vi "FL3001_simpleFFT.VI"() -> ()   [LabVIEW 2015]
uses:
  board.vis/Globals.vi
panel:
  in  "continuous":bool
  in  "exit":bool
  out "meanB":dbl=197.0 format="%0#.1f"
  out "tRMSB":dbl format="%0#.1f"
  out "meanA":dbl=9163.524137931034 format="%0#.1f"
  in  "TRMS Pix":u32=550
  out "Signal Cam 2":u16[](graph)
  in  "extTrig":bool
  in  "ext. trig. slope":enum32{"1", "2", "3"}(radio)
  out "tRMSA":dbl=7.44979324293522 format="%0#.1f"
  out "Measure ON":bool
  in  "no.of blocks (nob)":u32=1
  in  "block":u32(slide)=1 max=10 scale=0.9..1.0
  out "Signal Cam1":u16[](graph)=[9561, 9604, 0, 1, 0, 328, 0, 0, 9709, 10494, 10571, 10581, 10601, 10615, 10647, 10653, 10690, 10710, 10746, 10759, 10759, 10759, 10895, 10918, 10956, 10990, 11009, 11035, 11062, 11093, 11094, 11132, 11153, 11163, 11174, 11214, 11226, 11266, 11275, 11312, 11312, 11332, 11366, 11390, 11417, 11427, 11449, 11469, 11521, 11534, 11583, 11593, 11641, 11662, 11679, 11694, 11737, 11762, 11774, 11783, 11783, 11783, 11783, 11783, 11920, 11930, 11959, 11974, 11989, 12026, 12049, 12084, 12103, 12150, 12155, 12183, 12211, 12240, 12248, 12284, 12315, 12354, 12370, 12377, 12400, 12438, 12452, 12496, 12508, 12527, 12549, 12602, 12594, 12642, 12656, 12681, 12709, 12743, 12757, 12795, 12794, 12807, 12807, 12807, 12807, 12807, 12807, 12967, 12988, 13001, 13011, 13047, 13089, 13091, 13092, 13129, 13161, 13146, 13209, 13224, 13248, 13291, 13287, 13299, 13340, 13369, 13392, 13408, 13438, 13466, 13473, 13527, 13541, 13568, 13587, 13627, 13657, 13707, 13731, 13760, 13817, 13831, 13831, 13831, 13831, 13989, 14036, 14106, 14146, 14191, 14230, 14290, 14338, 14392, 14441, 14483, 14518, 14577, 14638, 14699, 14740, 14794, 14855, 14855, 14855, 15072, 15093, 15168, 15231, 15307, 15358, 15391, 15480, 15534, 15615, 15686, 15769, 15819, 15891, 15968, 16012, 16100, 16195, 16252, 16337, 16412, 16476, 16563, 16632, 16689, 16784, 16856, 16903, 16903, 17060, 17153, 17223, 17287, 17387, 17454, 17529, 17634, 17720, 17787, 17874, 17927, 17927, 18168, 18238, 18341, 18440, 18540, 18602, 18704, 18811, 18897, 18951, 19096, 19210, 19315, 19399, 19518, 19623, 19758, 19826, 19927, 19975, 19975, 20226, 20347, 20459, 20564, 20669, 20798, 20885, 20999, 21131, 21240, 21332, 21432, 21582, 21689, 21801, 21933, 22036, 22143, 22221, 22353, 22440, 22547, 22624, 22719, 22796, 22893, 22979, 23047, 23047, 23208, 23319, 23398, 23462, 23562, 23613, 23731, 23808, 23873, 23975, 24037, 24071, 24071, 24296, 24399, 24443, 24531, 24616, 24700, 24811, 24871, 24952, 25035, 25093, 25248, 25309, 25404, 25478, 25546, 25615, 25718, 25827, 25902, 25997, 26044, 26119, 26119, 26323, 26393, 26479, 26574, 26649, 26720, 26792, 26910, 27011, 27074, 27143, 27143, 27350, 27420, 27510, 27599, 27681, 27712, 27801, 27905, 28024, 28110, 28167, 28167, 28345, 28409, 28433, 28482, 28469, 28507, 28495, 28432, 28406, 28317, 28167, 28167, 28037, 27914, 27802, 27663, 27539, 27380, 27143, 27046, 26887, 26742, 26596, 26445, 26310, 26119, 26009, 25909, 25785, 25678, 25595, 25531, 25422, 25393, 25361, 25332, 25299, 25313, 25357, 25399, 25446, 25511, 25518, 25660, 25718, 25827, 25907, 25944, 25898, 25886, 25845, 25777, 25728, 25600, 25541, 25445, 25348, 25245, 25095, 25024, 24905, 24756, 24560, 24358, 24071, 23885, 23654, 23369, 23047, 22894, 22611, 22355, 22091, 21833, 21605, 21356, 21137, 20900, 20682, 20479, 20244, 19975, 19822, 19604, 19367, 19176, 18932, 18710, 18477, 18257, 17927, 17833, 17611, 17395, 17228, 16903, 16883, 16696, 16542, 16398, 16249, 16123, 15993, 15866, 15774, 15655, 15547, 15463, 15391, 15336, 15264, 15207, 15179, 15158, 15112, 15116, 15127, 15136, 15151, 15158, 15184, 15215, 15229, 15210, 15261, 15273, 15277, 15302, 15311, 15315, 15328, 15351, 15344, 15367, 15377, 15392, 15403, 15438, 15408, 15430, 15451, 15463, 15452, 15449, 15470, 15507, 15491, 15503, 15522, 15535, 15543, 8347, 8048, 8032, 8045, 8044, 8055, 8082, 8087, 8108, 8111, 8134, 8143, 8159, 8166, 8186, 8194, 8224, 8225, 8237, 8257, 8266, 8278, 8305, 8318, 8318, 8340, 8348, 8366, 8366, 8394, 8406, 8411, 8434, 8457, 8461, 8478, 8488, 8508, 8518, 8526, 8552, 8559, 8577, 8583, 8591, 8616, 8627, 8644, 8664, 8676, 8698, 8711, 8711, 8711, 8711, 8711, 8711, 8711, 8711, 8711, 8853, 8863, 8888, 8902, 8896, 8922, 8938, 8959, 8969, 8991, 9002, 9022, 9040, 9048, 9060, 9086, 9098, 9104, 9137, 9153, 9161, 9169, 9180, 9193, 9203, 9221, 9241, 9252, 9251, 9281, 9300, 9303, 9324, 9351, 9344, 9362, 9383, 9395, 9430, 9442, 9447, 9464, 9490, 9513, 9522, 9532, 9564]
  out "FREE \nRAM MB":dbl=27108.19140625
  out "BUILT-IN\nRAM MB":dbl=32640.29296875
  out "SEC":dbl=0.5
  out "MB RAM":dbl=0.54931640625
  in  "DAT in 10ns":u32
  in  "start":bool
  in  "sample":u32(slide)=328 max=3000 scale=0.9..500.0
  in  "no.of samples (nos)":u32=500
  in  "exposuretime[ms]":dbl=1.0 format="%.3f"
  # "press cont to stop, \nEsc to abort\nmeasurement"
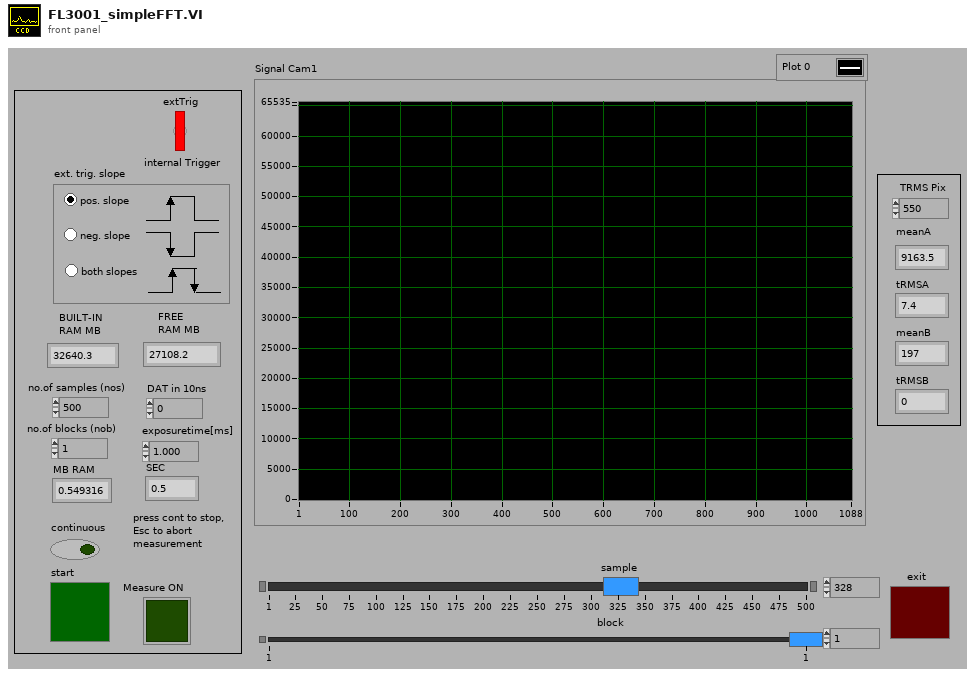
[diagram p1: front panel]
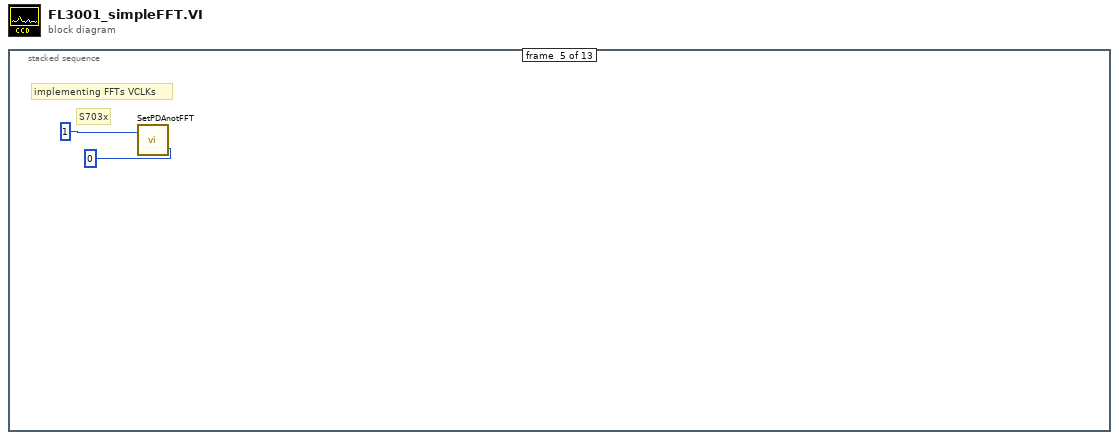
[diagram p0: block diagram]
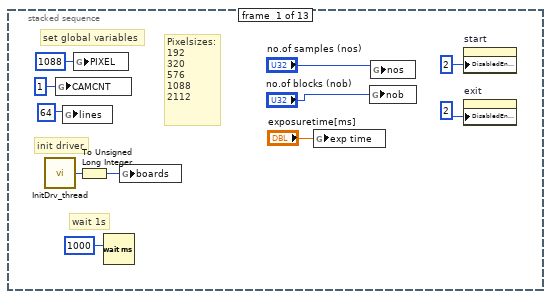
[diagram p2: hidden frame]
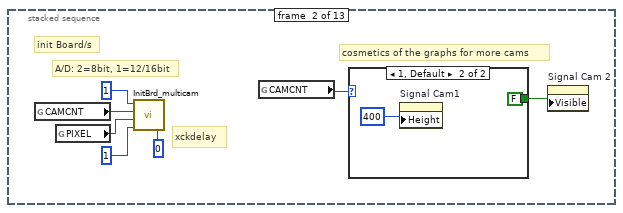
[diagram p3: hidden frame]
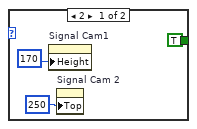
[diagram p4: hidden frame]
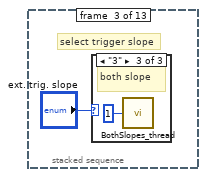
[diagram p5: hidden frame]
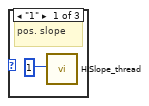
[diagram p6: hidden frame]
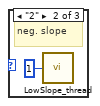
[diagram p7: hidden frame]
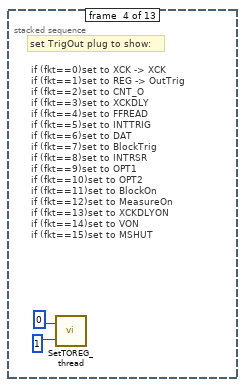
[diagram p8: hidden frame]
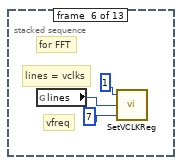
[diagram p9: hidden frame]
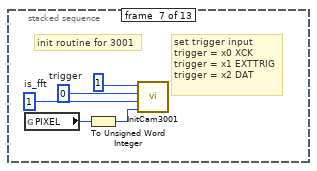
[diagram p10: hidden frame]
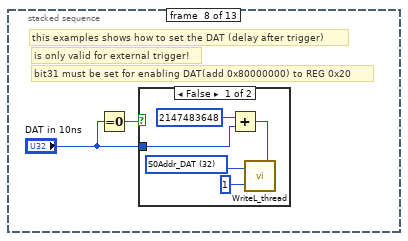
[diagram p11: hidden frame]
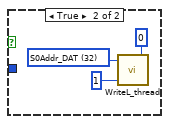
[diagram p12: hidden frame]
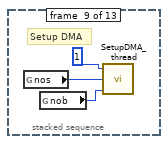
[diagram p13: hidden frame]
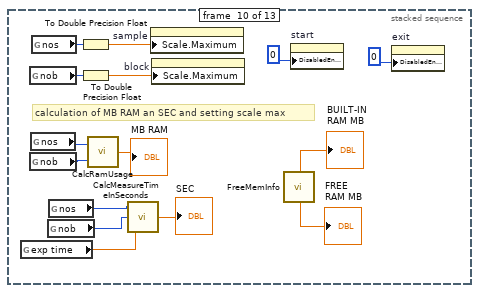
[diagram p14: hidden frame]
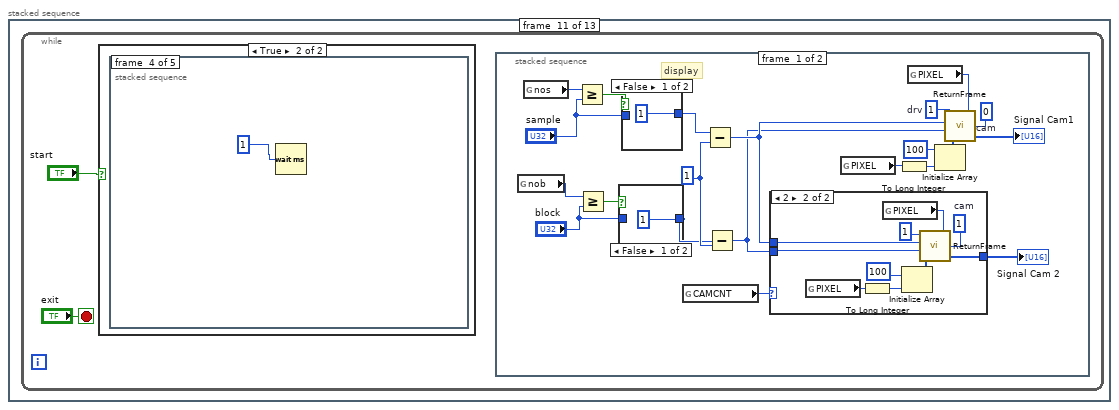
[diagram p15: hidden frame]
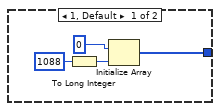
[diagram p16: hidden frame]
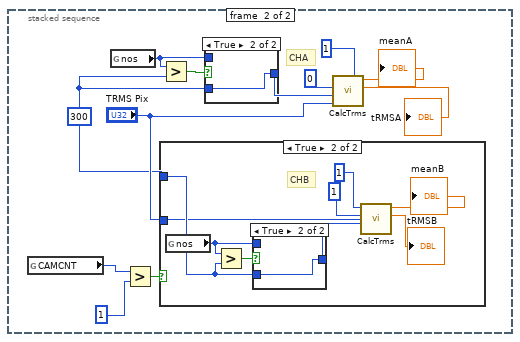
[diagram p19: hidden frame]
diagram:
  n1 = stacked-sequence {
    frame #0 {
      # "wait 1s"
      # "Pixelsizes:\n192\n320\n576\n1088\n2112"
      # "set global variables"
      # "init driver"
      n2 = call "InitDrv_thread.vi"() -> ("Boards"=w11:u8)  [unwired: 1 in]
      n3 = global write "Globals.vi" "CAMCNT"(u32 1) -> ()
      n4 = global write "Globals.vi" "lines"(u32 64) -> ()
      n5 = global write "Globals.vi" "PIXEL"(u32 1088) -> ()
      n6 = To Unsigned Long Integer(number=w11) -> (unsigned 32bit integer=w10:u32)
      n7 = Wait (ms)(milliseconds to wait=u32 1000) -> ()  [unwired: 1 out]
      n8 = global write "Globals.vi" "boards"(w10) -> ()
      n9 = global write "Globals.vi" "exp time"("exposuretime[ms]") -> ()
      n10 = global write "Globals.vi" "nob"("no.of blocks (nob)") -> ()
      n11 = global write "Globals.vi" "nos"("no.of samples (nos)") -> ()
      n12 = property on="start" class="Bool (strict)"("DisabledEnum"=u32 2) -> ()  [unwired: 2 in, 2 out]
      n13 = property on="exit" class="Bool (strict)"("DisabledEnum"=u32 2) -> ()  [unwired: 2 in, 2 out]
    }
    frame #1 {
      # "cosmetics of the graphs for more cams"
      # "xckdelay"
      # "init Board/s"
      # "A/D: 2=8bit, 1=12/16bit"
      n14 = global read "Globals.vi" "CAMCNT"() -> (w18:u32)
      n15 = global read "Globals.vi" "PIXEL"() -> (w16:u32)
      n16 = call "InitBrd_multicam.vi"("xckdly"=u32 0, "flag816"=u32 1, "pixel"=w16, "camcnt"=w18, "board_sel"=u32 1) -> ()  [unwired: 2 in]
      n17 = global read "Globals.vi" "CAMCNT"() -> (w12:u32)
      n18 = case shown="1, Default" w12 {
        tunnel: [TRUE FALSE] -> w13
        frame 2 {
          n19 = property on="Signal Cam1" class="WFGraph (strict)"("Height"=u32 170) -> ()  [unwired: 2 in, 2 out]
          n20 = property on="Signal Cam 2" class="WFGraph (strict)"("Top"=250) -> ()  [unwired: 2 in, 2 out]
        }
        frame 1, Default {
          n21 = property on="Signal Cam1" class="WFGraph (strict)"("Height"=u32 400) -> ()  [unwired: 2 in, 2 out]
        }
      }
      n22 = property on="Signal Cam 2" class="WFGraph (strict)"("Visible"=w13) -> ()  [unwired: 2 in, 2 out]
    }
    frame #2 {
      # "select trigger slope"
      n23 = case shown="\"3\"" "ext. trig. slope" {
        frame "1" {
          # "pos. slope"
          n24 = call "HiSlope_thread.vi"("board_sel"=u32 1) -> ()  [unwired: 1 in]
        }
        frame "2" {
          # "neg. slope"
          n25 = call "LowSlope_thread.vi"("board_sel"=u32 1) -> ()  [unwired: 1 in]
        }
        frame "3" {
          # "both slope"
          n26 = call "BothSlopes_thread.vi"("board_sel"=u32 1) -> ()  [unwired: 1 in]
        }
      }
    }
    frame #3 {
      # "if (fkt==0)set to XCK -> XCK\nif (fkt==1)set to REG -> OutTrig\nif (fkt==2)set to CNT_O\nif (fkt==3)set to XCKDLY\nif (fkt==4)set to FFREAD\nif (fkt==5)set to INTTRIG\nif (fkt==6)set to DAT\nif (fkt==7)set to BlockTrig\nif (fkt==8)set to INTRSR\nif (fkt==9)set to OPT1\nif (fkt==10)set to OPT2\nif (fkt==11)set to BlockOn\nif (fkt==12)set to MeasureOn\nif (fkt==13)set to XCKDLYON \nif (fkt==14)set to VON         \nif (fkt==15)set to MSHUT"
      # "set TrigOut plug to show:"
      n27 = call "SetTOREG_thread.vi"("board_sel"=u32 1, "fkt"=u8 0) -> ()  [unwired: 1 in]
    }
    frame #4 {
      # "S703x"
      # "implementing FFTs VCLKs"
      n28 = call "SetPDAnotFFT.vi"("set"=u8 0, "board_sel"=u32 1) -> ()  [unwired: 1 in]
    }
    frame #5 {
      # "vfreq"
      # "lines = vclks"
      # "for FFT"
      n29 = global read "Globals.vi" "lines"() -> (w34:u32)
      n30 = call "SetVCLKReg.vi"("vfreq"=u8 7, "lines"=w34, "board_sel"=u32 1) -> ()  [unwired: 1 in]
    }
    frame #6 {
      w35 = u16 1  # is_fft
      w36 = u16 0  # trigger
      # "set trigger input\ntrigger = x0 XCK\ntrigger = x1 EXTTRIG\ntrigger = x2 DAT"
      # "init routine for 3001"
      n31 = global read "Globals.vi" "PIXEL"() -> (w39:u32)
      n32 = To Unsigned Word Integer(number=w39) -> (unsigned 16bit integer=w37:u16)
      n33 = call "InitCam3001.vi"("pixel"=w37, "IS_FFT"=w35, "trigger_input"=w36, "drvno"=u32 1) -> ()  [unwired: 1 in]
    }
    frame #7 {
      # "bit31 must be set for enabling DAT(add 0x80000000) to REG 0x20"
      # "is only valid for external trigger!"
      # "this examples shows how to set the DAT (delay after trigger)"
      n34 = Equal To 0?(x="DAT in 10ns") -> (x = 0?=w41:bool)
      n35 = case shown="False" w41 {
        tunnel: "DAT in 10ns" -> [w45 _]
        frame False {
          w43 = u8 32 items=["S0Addr_CtrlA"=4, "S0Addr_CtrlB"=5, "S0Addr_CtrlC"=6, "S0Addr_XCKLL"=8, "S0Addr_XCKLH"=9, "S0Addr_XCKHL"=10, "S0Addr_XCKMSB"=11, "S0Addr_XCKCNTLL"=12, "S0Addr_XCKCNTLH"=13, "S0Addr_XCKCNTHL"=14, "S0Addr_XCKCNTMSB"=15, "S0Addr_PIXREGlow"=16, "S0Addr_PIXREGhigh"=17, "S0Addr_FREQREG"=18, "S0Addr_FF_FLAGS"=19, "S0Addr_FIFOCNT"=20, "S0Addr_VCLKCTRL"=24, "S0Addr_EBST"=28, "S0Addr_DAT"=32, "S0Addr_EC"=36, "S0Addr_TOR"=40, "S0Addr_ARREG"=44, "S0Addr_GIOREG"=48, "S0Addr_DELAYEC"=52, "S0Addr_IRQREG"=56, "S0Addr_PCI"=60]
          n36 = Add(x=u32 2147483648, y=w45) -> (x+y=w44:u32)
          n37 = call "WriteL_thread.vi"("val"=w44, "board_sel"=u32 1, "offset"=w43) -> ()
        }
        frame True {
          w48 = u8 32 items=["S0Addr_CtrlA"=4, "S0Addr_CtrlB"=5, "S0Addr_CtrlC"=6, "S0Addr_XCKLL"=8, "S0Addr_XCKLH"=9, "S0Addr_XCKHL"=10, "S0Addr_XCKMSB"=11, "S0Addr_XCKCNTLL"=12, "S0Addr_XCKCNTLH"=13, "S0Addr_XCKCNTHL"=14, "S0Addr_XCKCNTMSB"=15, "S0Addr_PIXREGlow"=16, "S0Addr_PIXREGhigh"=17, "S0Addr_FREQREG"=18, "S0Addr_FF_FLAGS"=19, "S0Addr_FIFOCNT"=20, "S0Addr_VCLKCTRL"=24, "S0Addr_EBST"=28, "S0Addr_DAT"=32, "S0Addr_EC"=36, "S0Addr_TOR"=40, "S0Addr_ARREG"=44, "S0Addr_GIOREG"=48, "S0Addr_DELAYEC"=52, "S0Addr_IRQREG"=56, "S0Addr_PCI"=60]
          n38 = call "WriteL_thread.vi"("val"=u32 0, "board_sel"=u32 1, "offset"=w48) -> ()
        }
      }
    }
    frame #8 {
      # "Setup DMA"
      n39 = global read "Globals.vi" "nos"() -> (w52:u32)
      n40 = global read "Globals.vi" "nob"() -> (w51:u32)
      n41 = call "SetupDMA_thread.vi"("blocks"=w51, "nos"=w52, "Board_sel"=u32 1) -> ()  [unwired: 2 in]
    }
    frame #9 {
      # "calculation of MB RAM an SEC and setting scale max"
      n42 = global read "Globals.vi" "exp time"() -> (w54:dbl)
      n43 = global read "Globals.vi" "nob"() -> (w63:u32)
      n44 = global read "Globals.vi" "nob"() -> (w57:u32)
      n45 = global read "Globals.vi" "nos"() -> (w58:u32)
      n46 = global read "Globals.vi" "nos"() -> (w65:u32)
      n47 = global read "Globals.vi" "nob"() -> (w55:u32)
      n48 = global read "Globals.vi" "nos"() -> (w56:u32)
      n49 = To Double Precision Float(number=w65) -> (double precision float=w64:dbl)
      n50 = To Double Precision Float(number=w63) -> (double precision float=w62:dbl)
      n51 = call "CalcRamUsage.vi"("nob"=w57, "nos"=w58) -> ("ramUsage"=→"MB RAM":dbl)
      n52 = call "CalcMeasureTimeInSeconds.vi"("exposure_time_in_ms"=w54, "nob"=w55, "nos"=w56) -> ("measureTimeInSeconds"=→"SEC":dbl)
      n53 = property on="sample" class="Slide (strict)"("Scale.Maximum"=w64) -> ()  [unwired: 2 in, 2 out]
      n54 = property on="block" class="Slide (strict)"("Scale.Maximum"=w62) -> ()  [unwired: 2 in, 2 out]
      n55 = call "FreeMemInfo.vi"() -> ("PhysicalSpace"=→"BUILT-IN\nRAM MB":dbl, "PhysicalFreeSpace"=→"FREE \nRAM MB":dbl)  [unwired: 1 in]
      n56 = property on="start" class="Bool (strict)"("DisabledEnum"=u32 0) -> ()  [unwired: 2 in, 2 out]
      n57 = property on="exit" class="Bool (strict)"("DisabledEnum"=u32 0) -> ()  [unwired: 2 in, 2 out]
    }
    frame #10 {
      n58 = while {
        stop <- "exit" stop-if-true
        n59 = case shown="True" "start" {
          frame False {
          }
          frame True {
            n60 = stacked-sequence {
              frame #0 {
                # "ext. block trig\n0: internal: Space\n1: PCI \"I\"\n2: S1\n3: S2"
                # "block trigger (depreciated, keep 0)\n0: internal -> next block is started immediately \n1: external -> all blocks on one trigger (via DLL)\n2: external -> one block per trigger (via DLL)"
                # "start measurement"
                n61 = global read "Globals.vi" "exp time"() -> (w137:dbl)
                n62 = Multiply(x=1000.0, y=w137) -> (x*y=w135:dbl)
                n63 = To Unsigned Long Integer(number=w135) -> (unsigned 32bit integer=w142:u32)
                n64 = case shown="True" "extTrig" {
                  tunnel: [u8 0 u8 1] -> w140
                  frame False {
                  }
                  frame True {
                  }
                }
                n65 = call "ReadFFLoop_thread.vi"("board_sel"=u32 1, "exptus"=w142, "ExtTrig"=w140, "btrig_ch"=u8 3, "blocktrigger"=u8 0) -> ()
              }
              frame #1 {
                n66 = while {
                  stop <- w147 stop-if-true
                  n67 = call "ReadB.vi"("Offset"=u32 64, "board_sel"=u32 1) -> ("Data 2"=w150:u8, "Data 1"=w151:u8)
                  n68 = call "Elapsed Time"("Time Target (s)"=1.0) -> ("Time has Elapsed"=w146:bool)  [unwired: 11 in, 7 out]
                  n69 = Or(x=w151, y=w150) -> (x .or. y?=w152:u8)
                  n70 = Number To Boolean Array(number=w152) -> (Boolean array=w154:bool[])
                  n71 = Index Array(array=w154, index=5) -> (element=w145:bool)
                  n72 = property on="Measure ON" class="Bool (strict)"("Value"=w145) -> ()  [unwired: 2 in, 2 out]
                  n73 = Or(x=w145, y=w146) -> (x .or. y?=w147:bool)
                }
              }
              frame #2 {
                n74 = while {
                  stop <- w156 continue-if-true
                  n75 = call "ReadB.vi"("Offset"=u32 64, "board_sel"=u32 1) -> ("Data 2"=w158:u8, "Data 1"=w159:u8)
                  n76 = Or(x=w159, y=w158) -> (x .or. y?=w160:u8)
                  n77 = Number To Boolean Array(number=w160) -> (Boolean array=w162:bool[])
                  n78 = Index Array(array=w162, index=5) -> (element=w156:bool)
                  "Measure ON" <- w156
                }
              }
              frame #3 {
                n79 = Wait (ms)(milliseconds to wait=u32 1) -> ()  [unwired: 1 out]
              }
              frame #4 {
                n80 = case shown="True" "continuous" {
                  frame False {
                    n81 = property on="start" class="Bool (strict)"("Value"=FALSE) -> ()  [unwired: 2 in, 2 out]
                  }
                  frame True {
                    n82 = property on="start" class="Bool (strict)"("Value"=TRUE) -> ()  [unwired: 2 in, 2 out]
                  }
                }
              }
            }
          }
        }
        n83 = stacked-sequence {
          frame #0 {
            w73 = u16 0  # cam
            w76 = u32 1  # drv
            w90 = u32 1
            # "display"
            n84 = global read "Globals.vi" "nob"() -> (w84:u32)
            n85 = global read "Globals.vi" "nos"() -> (w89:u32)
            n86 = Greater Or Equal?(x=w89, y="sample") -> (x >= y?=w82:bool)
            n87 = Greater Or Equal?(x=w84, y="block") -> (x >= y?=w81:bool)
            n88 = case shown="False" w81 {
              tunnel: [u32 1 w106] -> w86
              tunnel: "block" -> [_ w106]
              frame False {
              }
              frame True {
              }
            }
            n89 = case shown="False" w82 {
              tunnel: [u32 1 w108] -> w88
              tunnel: "sample" -> [_ w108]
              frame False {
              }
              frame True {
              }
            }
            n90 = global read "Globals.vi" "CAMCNT"() -> (w83:u32)
            n91 = Subtract(x=w88, y=w90) -> (x-y=w72:u32)
            n92 = Subtract(x=w86, y=w90) -> (x-y=w71:u32)
            n93 = case shown="2" w83 {
              tunnel: w71 -> [_ w98]
              tunnel: w72 -> [_ w96]
              tunnel: [w91 w99] -> w80
              frame 1, Default {
                n94 = To Long Integer(number=u16 1088) -> (32bit integer=w92:i32)
                n95 = Initialize Array(u16 0, w92) -> (w91:u16[])
              }
              frame 2 {
                w97 = u16 1  # cam
                n96 = global read "Globals.vi" "PIXEL"() -> (w100:u32)
                n97 = To Long Integer(number=w100) -> (32bit integer=w101:i32)
                n98 = global read "Globals.vi" "PIXEL"() -> (w95:u32)
                n99 = Initialize Array(u16 100, w101) -> (w102:u16[])
                n100 = call "ReturnFrame.vi"("curr_cam"=w97, "length"=w95, "Data Values In"=w102, "curr_nob"=w98, "curr_nos"=w96, "Drv"=u32 1) -> ("Data Values Out"=w99:u16[])
              }
            }
            "Signal Cam 2" <- w80
            n101 = global read "Globals.vi" "PIXEL"() -> (w79:u32)
            n102 = To Long Integer(number=w79) -> (32bit integer=w78:i32)
            n103 = global read "Globals.vi" "PIXEL"() -> (w70:u32)
            n104 = Initialize Array(u16 100, w78) -> (w74:u16[])
            n105 = call "ReturnFrame.vi"("curr_cam"=w73, "length"=w70, "Data Values In"=w74, "curr_nob"=w71, "curr_nos"=w72, "Drv"=w76) -> ("Data Values Out"=→"Signal Cam1":u16[])
          }
          frame #1 {
            w115 = u32 300
            # "CHA"
            n106 = global read "Globals.vi" "CAMCNT"() -> (w117:u32)
            n107 = global read "Globals.vi" "nos"() -> (w111:u32)
            n108 = Greater?(x=w117, y=u32 1) -> (0:w119:bool)
            n109 = case shown="True" w119 {
              tunnel: w115 -> [_ w124]
              tunnel: "TRMS Pix" -> [_ w123]
              frame False {
              }
              frame True {
                # "CHB"
                n110 = global read "Globals.vi" "nos"() -> (w127:u32)
                n111 = Greater?(x=w127, y=w124) -> (0:w129:bool)
                n112 = case shown="True" w129 {
                  tunnel: [w130 w131] -> w128
                  tunnel: w124 -> [_ w131]
                  tunnel: w127 -> [w130 _]
                  frame False {
                  }
                  frame True {
                  }
                }
                n113 = call "CalcTrms.vi"("TRMSpix"=w123, "scans"=w128, "CAMpos"=u16 1, "board_sel"=u32 1) -> ("TRMS 1"=→"tRMSB":dbl, "mean 1"=→"meanB":dbl)  [unwired: 2 out]
              }
            }
            n114 = Greater?(x=w111, y=w115) -> (0:w109:bool)
            n115 = case shown="True" w109 {
              tunnel: [w132 w133] -> w110
              tunnel: w115 -> [_ w133]
              tunnel: w111 -> [w132 _]
              frame False {
              }
              frame True {
              }
            }
            n116 = call "CalcTrms.vi"("TRMSpix"="TRMS Pix", "scans"=w110, "CAMpos"=u16 0, "board_sel"=u32 1) -> ("TRMS 1"=→"tRMSA":dbl, "mean 1"=→"meanA":dbl)  [unwired: 2 out]
          }
        }
      }
    }
    frame #11 {
      n117 = call "FFStop.vi"() -> ()  [unwired: 1 in]
    }
    frame #12 {
      # "exit"
      # "do not omit, or next call of driver will go wrong."
      n118 = call "Exit.vi"("board_sel"=u32 1) -> ()  [unwired: 1 in]
    }
  }
